vi "Teleop.vi"(10 "Match Info":T1={"Autonomous Elapsed Seconds"=0.0, "TeleOp Elapsed Seconds"=0.0, "Disabled Elapsed Seconds"=0.0, "Visited Autonomous"=FALSE, "Visited TeleOp"=FALSE, "Visited Disabled"=FALSE, "Autonomous Settings"={"Autonomous Style"=enum."Independent", "VI Refnum"=refnum}}, 11 "Call Context":T2) -> ()   [LabVIEW 2023]
doc: "This VI is called for each TeleOp packet received from the DS where the robot is not disabled. It is often used to read from the joysticks and update I/O or to update setpoints for timed control loops. It should complete and return within 20 milliseconds or it may miss DS packets."
uses:
  <vilib>/Rock Robotics/WPI/DriverStation/WPI_DriverStationDerivedRobotMode.ctl
  <vilib>/Rock Robotics/WPI/DriverStation/WPI_DriverStationMatch Info.ctl
  <vilib>/Rock Robotics/Network Tables/NT Read Boolean.vi
  <vilib>/Rock Robotics/Network Tables/NT Read Number.vi
  <vilib>/Rock Robotics/WPI/Utilities/WPI_GetSetVariantRefNum.vi
  Robot Global Data.vi
  <vilib>/addons/control/pid/pid.llb/PID Output Rate Limiter (DBL).vi
  <vilib>/Rock Robotics/Network Tables/NT Write Numeric Array.vi
  <vilib>/addons/control/pid/NI_PID_pid.lvlib
  <vilib>/Rock Robotics/Network Tables/NT Write Boolean Array.vi
panel:
  out "Sensor Position 2":dbl
  out "Sensor Position":dbl
  in  "output rate (EGU/min) 2":dbl=1.0 format="%.2f"
  in  "output rate (EGU/min)":dbl=1.0 format="%.2f"
  out "Sample Slider 0":dbl(slide) scale=0.0..5.0
  out "Sample Boolean 1":bool
  out "Sample Boolean 0":bool
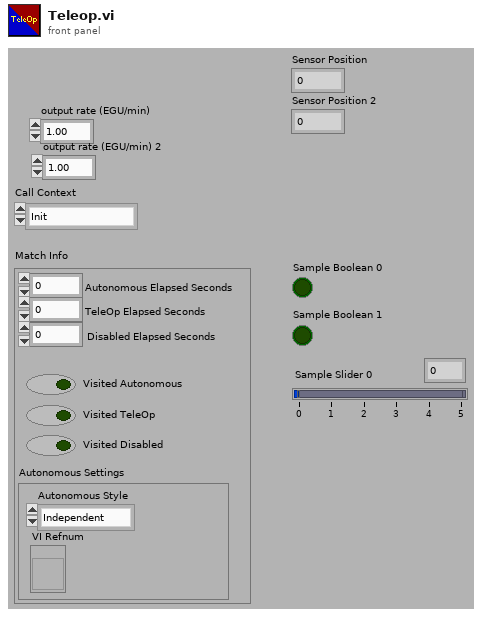
[diagram p1: front panel]
types:
  T1 = typedef "WPI_DriverStationMatch Info.ctl" = cluster{"Autonomous Elapsed Seconds":dbl, "TeleOp Elapsed Seconds":dbl, "Disabled Elapsed Seconds":dbl, "Visited Autonomous":bool, "Visited TeleOp":bool, "Visited Disabled":bool, "Autonomous Settings":cluster{"Autonomous Style":enum16{"Iterative", "Independent"}, "VI Refnum":refnum<vi>}}
  T2 = typedef "WPI_DriverStationDerivedRobotMode.ctl" = enum16{"Init", "Execute", "Stop"}
  T3 = typedef "WPI_JoystickDevRef.ctl" = cluster{"Device":T4}
  T4 = typedef "WPI_JoystickDeviceEnum.ctl" = enum16{"USB 0", "USB 1", "USB 2", "USB 3", "USB 4", "USB 5"}
  T5 = typedef "WPI_RobotDriveDevRef.ctl" = cluster{"DevStatus":errorcluster, "Motors[]":T6[], "Square Inputs":bool, "Max Output":dbl}
  T6 = typedef "WPI_MotorControlDeviceRef.ctl" = cluster{"DeviceStatus":errorcluster, "Type":T7, "PWM":cluster{"PWM Channel":T8, "DeadBand":T9}, "CAN":cluster{"Device Number":u8, "SetOutput VI Ref":variant, "GetOutput VI Ref":variant, "Enable VI Ref":variant, "Disable VI Ref":variant, "Data":variant}, "Invert":bool, "DIO PWM":cluster{"PWM \"Enable\" Channel":T8, "DIOChannel":T10, "PWM Rate":dbl}}
  T7 = typedef "WPI_MotorControlType.ctl" = enum16{"PWM", "CAN", "DIO PWM"}
  T8 = typedef "FPGA_DIOPWMChannel.ctl" = enum8{"PWM 0", "PWM 1", "PWM 2", "PWM 3", "PWM 4", "PWM 5", "PWM 6", "PWM 7", "PWM 8", "PWM 9", "PWM MXP 0", "PWM MXP 1", "PWM MXP 2", "PWM MXP 3", "PWM MXP 4", "PWM MXP 5", "PWM MXP 6", "PWM MXP 7", "PWM MXP 8", "PWM MXP 9", "Invalid"}
  T9 = typedef "WPI_PWMDeadband.ctl" = cluster{"Name":string, "maxPositivePwm":i32, "minPositivePwm":i32, "centerPwm":i32, "maxNegativePwm":i32, "minNegativePwm":i32, "angularRange":u16}
  T10 = typedef "FPGA_DIOChannel.ctl" = enum8{"DIO 0", "DIO 1", "DIO 2", "DIO 3", "DIO 4", "DIO 5", "DIO 6", "DIO 7", "DIO 8", "DIO 9", "DIO MXP 0", "DIO MXP 1", "DIO MXP 2", "DIO MXP 3", "DIO MXP 4", "DIO MXP 5", "DIO MXP 6", "DIO MXP 7", "DIO MXP 8", "DIO MXP 9", "DIO MXP 10", "DIO MXP 11", "DIO MXP 12", "DIO MXP 13", "DIO MXP 14", "DIO MXP 15", "SPI Port CS1", "SPI Port CS2", "SPI Port CS3", "SPI Port MISO", "SPI Port MOSI", "Invalid"}
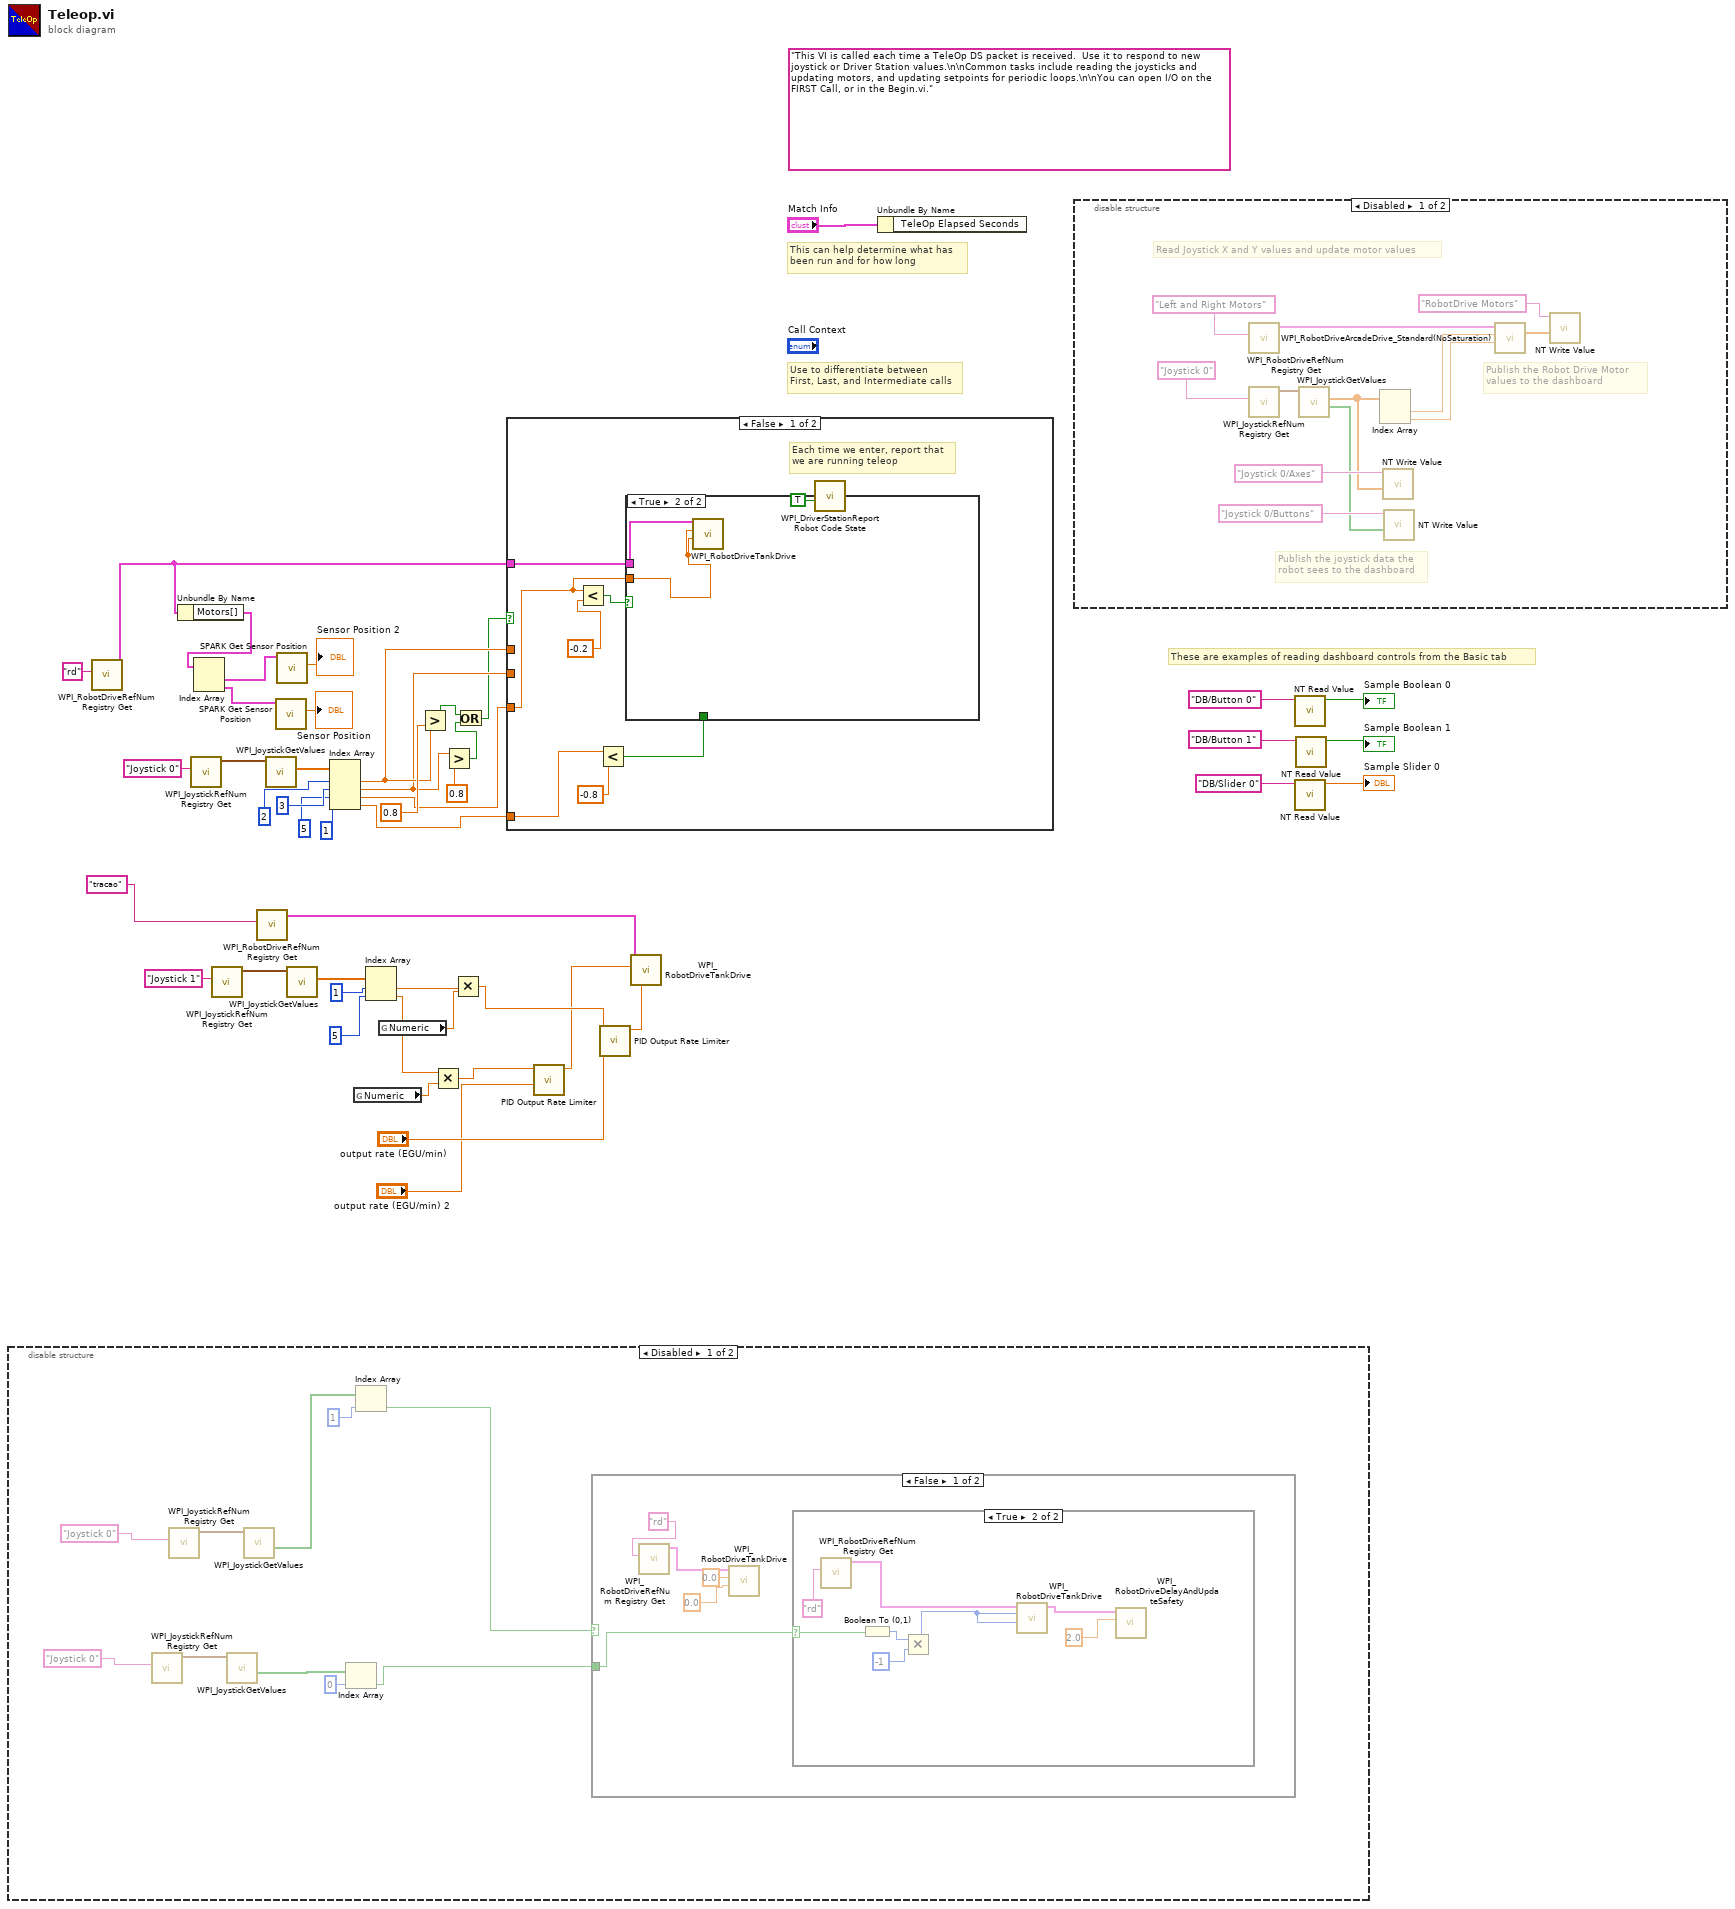
[diagram p0: block diagram]
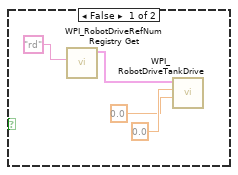
[diagram p2: hidden frame]
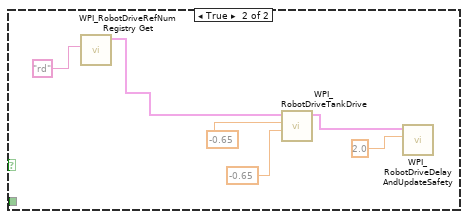
[diagram p3: hidden frame]
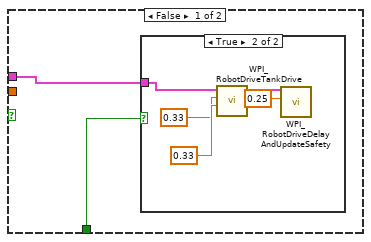
[diagram p5: hidden frame]
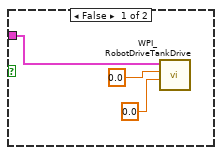
[diagram p6: hidden frame]
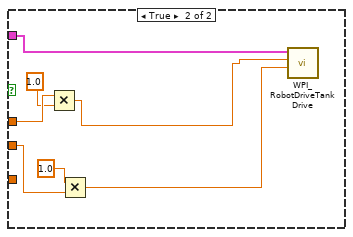
[diagram p7: hidden frame]
diagram:
  (unwired) "This VI is called each time a TeleOp DS packet is received.  Use it to respond to new joystick or Driver Station values.\n\nCommon tasks include reading the joysticks and updating motors, and updating setpoints for periodic loops.\n\nYou can open I/O on the FIRST Call, or in the Begin.vi."
  # "These are examples of reading dashboard controls from the Basic tab"
  # "Each time we enter, report that\nwe are running teleop"
  # "Use to differentiate between\nFirst, Last, and Intermediate calls"
  # "This can help determine what has\nbeen run and for how long"
  n1 = disable-structure shown="Disabled" {
    frame Disabled {
      n2 = call <vilib>:"WPI_JoystickRefNum Registry Get.vi"("refnum name"="Joystick 0") -> ("JoystickDevRef"=w53:T3)  [unwired: 9 in, 1 out]
      n3 = call <vilib>:"WPI_JoystickRefNum Registry Get.vi"("refnum name"="Joystick 0") -> ("JoystickDevRef"=w57:T3)  [unwired: 9 in, 1 out]
      n4 = call <vilib>:"WPI_JoystickGetValues.vi"("JoystickDevRef"=w53) -> ("Buttons"=w51:bool[])  [unwired: 6 in, 4 out]
      n5 = call <vilib>:"WPI_JoystickGetValues.vi"("JoystickDevRef"=w57) -> ("Buttons"=w56:bool[])  [unwired: 6 in, 4 out]
      n6 = Index Array(array=w51, index=0) -> (element=w49:bool)
      n7 = Index Array(array=w56, index=1) -> (element=w55:bool)
      n8 = case shown="False" w55 {
        tunnel: w49 -> [w63 _]
        frame False {
          n9 = call <vilib>:"WPI_RobotDriveRefNum Registry Get.vi"("refnum name"="rd") -> ("RobotDriveDevRef"=w61:T5)  [unwired: 9 in, 1 out]
          n10 = call <vilib>:"WPI_RobotDriveTankDrive.vi"("Right axis value"=0.0 ("Left axis value"), "Left axis value"=0.0, "RobotDriveDevRef"=w61) -> ()  [unwired: 6 in, 3 out]
          n11 = case shown="True" w63 {
            selector: w63 -> [_ w75]
            frame False {
              n12 = call <vilib>:"WPI_RobotDriveRefNum Registry Get.vi"("refnum name"="rd") -> ("RobotDriveDevRef"=w64:T5)  [unwired: 9 in, 1 out]
              n13 = call <vilib>:"WPI_RobotDriveTankDrive.vi"("Right axis value"=0.0 ("Left axis value"), "Left axis value"=0.0, "RobotDriveDevRef"=w64) -> ()  [unwired: 6 in, 3 out]
            }
            frame True {
              n14 = call <vilib>:"WPI_RobotDriveRefNum Registry Get.vi"("refnum name"="rd") -> ("RobotDriveDevRef"=w69:T5)  [unwired: 9 in, 1 out]
              n15 = Boolean To (0,1)(Boolean=w75) -> (0, 1=w72:i16)
              n16 = Multiply(x=w72, y=i16 -1) -> (x*y=w70:i16)
              n17 = call <vilib>:"WPI_RobotDriveTankDrive.vi"("Right axis value"=w70, "Left axis value"=w70, "RobotDriveDevRef"=w69) -> ("RobotDriveDevRef"=w74:T5)  [unwired: 6 in, 2 out]
              n18 = call <vilib>:"WPI_RobotDriveDelayAndUpdateSafety.vi"("Delay (s)"=2.0, "RobotDriveDevRef"=w74) -> ()  [unwired: 8 in, 2 out]
            }
          }
        }
        frame True {
          n19 = call <vilib>:"WPI_RobotDriveRefNum Registry Get.vi"("refnum name"="rd") -> ("RobotDriveDevRef"=w76:T5)  [unwired: 9 in, 1 out]
          n20 = call <vilib>:"WPI_RobotDriveTankDrive.vi"("Right axis value"=-0.65 ("Left axis value"), "Left axis value"=-0.65, "RobotDriveDevRef"=w76) -> ("RobotDriveDevRef"=w79:T5)  [unwired: 6 in, 2 out]
          n21 = call <vilib>:"WPI_RobotDriveDelayAndUpdateSafety.vi"("Delay (s)"=2.0, "RobotDriveDevRef"=w79) -> ()  [unwired: 8 in, 2 out]
        }
      }
    }
    frame Enabled {
    }
  }
  n22 = call <vilib>:"WPI_RobotDriveRefNum Registry Get.vi"("refnum name"="rd") -> ("RobotDriveDevRef"=w6:T5)  [unwired: 9 in, 1 out]
  n23 = Unbundle By Name(w6) -> ("Motors[]"=w5:T6[])
  n24 = call <vilib>:"WPI_JoystickRefNum Registry Get.vi"("refnum name"="Joystick 0") -> ("JoystickDevRef"=w38:T3)  [unwired: 9 in, 1 out]
  n25 = Index Array(array=w5) -> (element #1=w4:T6, element #2=w3:T6)  [unwired: 2 in]
  n26 = call <vilib>:"WPI_JoystickRefNum Registry Get.vi"("refnum name"="Joystick 1") -> ("JoystickDevRef"=w22:T3)  [unwired: 9 in, 1 out]
  n27 = call <vilib>:"WPI_RobotDriveRefNum Registry Get.vi"("refnum name"="tracao") -> ("RobotDriveDevRef"=w15:T5)  [unwired: 9 in, 1 out]
  n28 = call <vilib>:"WPI_JoystickGetValues.vi"("JoystickDevRef"=w38) -> ("Axes"=w39:dbl[])  [unwired: 6 in, 4 out]
  n29 = call <vilib>:"SPARK Get Sensor Position.vi"("MotorControlDevRef in"=w3) -> ("Sensor Position"=→"Sensor Position":dbl)  [unwired: 7 in, 3 out]
  n30 = call <vilib>:"SPARK Get Sensor Position.vi"("MotorControlDevRef in"=w4) -> ("Sensor Position"=→"Sensor Position 2":dbl)  [unwired: 7 in, 3 out]
  n31 = call <vilib>:"WPI_JoystickGetValues.vi"("JoystickDevRef"=w22) -> ("Axes"=w18:dbl[])  [unwired: 6 in, 4 out]
  n32 = Index Array(array=w39, index #1=2 ("index"), index #2=3 ("index"), index #3=5 ("index"), index #4=1 ("index")) -> (element #1=w33:dbl, element #2=w29:dbl, element #3=w31:dbl, element #4=w24:dbl)
  n33 = global read "Robot Global Data.vi" "Numeric"() -> (w7:dbl)
  n34 = Index Array(array=w18, index #1=1 ("index"), index #2=5 ("index")) -> (element #1=w12:dbl, element #2=w14:dbl)
  n35 = global read "Robot Global Data.vi" "Numeric"() -> (w8:dbl)
  n36 = Greater?(x=w33, y=0.8) -> (0:w30:bool)
  n37 = Multiply(x=w14, y=w7) -> (x*y=w13:dbl)
  n38 = Greater?(x=w29, y=0.8) -> (0:w27:bool)
  n39 = Multiply(x=w12, y=w8) -> (x*y=w11:dbl)
  n40 = Or(x=w30, y=w27) -> (x .or. y?=w26:bool)
  n41 = case shown="False" w26 {
    tunnel: w6 -> [w86 w107]
    tunnel: w33 -> [_ w106]
    tunnel: w29 -> [_ w103]
    tunnel: w31 -> [w85 _]
    tunnel: w24 -> [w84 _]
    frame False {
      n42 = Less?(x=w85, y=-0.2) -> (x < y?=w87:bool)
      n43 = Less?(x=w84, y=-0.8) -> (x < y?=w82:bool)
      n44 = case shown="True" w87 {
        tunnel: w86 -> [w89 w100]
        tunnel: w85 -> [_ w99]
        tunnel: w82 -> [w90 _]
        frame False {
          n45 = case shown="True" w90 {
            tunnel: w89 -> [w91 w96]
            frame False {
              n46 = call <vilib>:"WPI_RobotDriveTankDrive.vi"("Right axis value"=0.0 ("Left axis value"), "Left axis value"=0.0, "RobotDriveDevRef"=w91) -> ()  [unwired: 6 in, 3 out]
            }
            frame True {
              n47 = call <vilib>:"WPI_RobotDriveTankDrive.vi"("Right axis value"=0.33 ("Left axis value"), "Left axis value"=0.33, "RobotDriveDevRef"=w96) -> ("RobotDriveDevRef"=w95:T5)  [unwired: 6 in, 2 out]
              n48 = call <vilib>:"WPI_RobotDriveDelayAndUpdateSafety.vi"("Delay (s)"=0.25, "RobotDriveDevRef"=w95) -> ()  [unwired: 8 in, 2 out]
            }
          }
        }
        frame True {
          n49 = call <vilib>:"WPI_RobotDriveTankDrive.vi"("Right axis value"=w99, "Left axis value"=w99, "RobotDriveDevRef"=w100) -> ()  [unwired: 6 in, 3 out]
        }
      }
    }
    frame True {
      n50 = Multiply(x=w106, y=1.0) -> (x*y=w104:dbl)
      n51 = Multiply(x=1.0 ("y"), y=w103) -> (x*y=w101:dbl)
      n52 = call <vilib>:"WPI_RobotDriveTankDrive.vi"("Right axis value"=w101, "Left axis value"=w104, "RobotDriveDevRef"=w107) -> ()  [unwired: 6 in, 3 out]
    }
  }
  n53 = call-poly <vilib>:"PID Output Rate Limiter.vi"("output rate (EGU/min)"="output rate (EGU/min) 2", "input (controller output)"=w13) -> ("output"=w10:dbl)  [unwired: 6 in, 1 out]
  n54 = call-poly <vilib>:"PID Output Rate Limiter.vi"("output rate (EGU/min)"="output rate (EGU/min)", "input (controller output)"=w11) -> ("output"=w9:dbl)  [unwired: 6 in, 1 out]
  n55 = call <vilib>:"WPI_RobotDriveTankDrive.vi"("Right axis value"=w9, "Left axis value"=w10, "RobotDriveDevRef"=w15) -> ()  [unwired: 6 in, 3 out]
  n56 = call <vilib>:"WPI_DriverStationReport Robot Code State.vi"("TeleOp"=TRUE ("Autonomous")) -> ()  [unwired: 10 in, 1 out]
  n57 = Unbundle By Name("Match Info") -> ()  [unwired: 1 out]
  n58 = disable-structure shown="Disabled" {
    frame Disabled {
      # "Publish the Robot Drive Motor\nvalues to the dashboard"
      # "Publish the joystick data the\nrobot sees to the dashboard"
      # "Read Joystick X and Y values and update motor values"
      n59 = call <vilib>:"WPI_RobotDriveRefNum Registry Get.vi"("refnum name"="Left and Right Motors") -> ("RobotDriveDevRef"=w118:T5)  [unwired: 1 in, 9 out]
      n60 = call <vilib>:"WPI_JoystickRefNum Registry Get.vi"("refnum name"="Joystick 0") -> ("JoystickDevRef"=w115:T3)  [unwired: 1 in, 9 out]
      n61 = call <vilib>:"WPI_JoystickGetValues.vi"("JoystickDevRef"=w115) -> ("Buttons"=w110:bool[], "Axes"=w111:dbl[])  [unwired: 6 in, 3 out]
      n62 = Index Array(array=w111) -> (element #1=w117:dbl, element #2=w114:dbl)  [unwired: 2 in]
      n63 = call-poly <vilib>:"NT Write Value.vi"("value"=w111, "name"="Joystick 0/Axes" ("Name")) -> ()  [unwired: 9 in, 1 out]
      n64 = call-poly <vilib>:"NT Write Value.vi"("value"=w110, "name"="Joystick 0/Buttons" ("Name")) -> ()  [unwired: 9 in, 1 out]
      n65 = call <vilib>:"WPI_RobotDriveArcadeDrive_Standard(NoSaturation).vi"("Y axis value"=w114, "X axis value"=w117, "RobotDriveDevRef"=w118) -> ("Motor Values"=w109:dbl[])  [unwired: 1 in, 7 out]
      n66 = call-poly <vilib>:"NT Write Value.vi"("value"=w109, "name"="RobotDrive Motors" ("Name")) -> ()  [unwired: 9 in, 1 out]
    }
    frame Enabled {
    }
  }
  n67 = call-poly <vilib>:"NT Read Value.vi"("name"="DB/Button 0" ("refnum name")) -> ("value"=→"Sample Boolean 0":bool)  [unwired: 8 in, 2 out]
  n68 = call-poly <vilib>:"NT Read Value.vi"("name"="DB/Slider 0" ("refnum name")) -> ("value"=→"Sample Slider 0":dbl)  [unwired: 8 in, 2 out]
  n69 = call-poly <vilib>:"NT Read Value.vi"("name"="DB/Button 1" ("refnum name")) -> ("value"=→"Sample Boolean 1":bool)  [unwired: 8 in, 2 out]
